vi "Replace-PointOnBody-Dimension.vi"(6 "Add?":bool, 8 "Dimension":dbl, 9 "DimensionIndex":i32, 11 "Point":T1={"Coord4"=[0.0, 0.0, 0.0, 1.0], "ID"=0}) -> (3 "Point 2":T1={"Coord4"=[0.0, 0.0, 0.0, 1.0], "ID"=0})   [LabVIEW 2016, in "CAlex2.lvclass"]
uses:
  CAlex2.lvclass
  SerialChain/TypeDef/PointOnBody.ctl
  SerialChain/SerialChain.lvclass
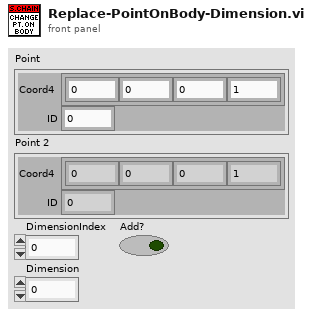
[diagram p1: front panel]
types:
  T1 = typedef "SerialChain.lvclass/PointOnBody.ctl" = cluster{"Coord4":dbl[], "ID":i32}
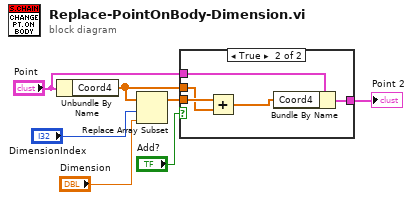
[diagram p0: block diagram]
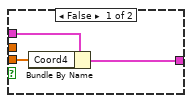
[diagram p2: hidden frame]
diagram:
  n1 = Unbundle By Name("Point") -> ("Coord4"=w1:dbl[])
  n2 = Replace Array Subset(array=w1, new element="Dimension", index="DimensionIndex") -> (w4:dbl[])
  n3 = case shown="True" "Add?" {
    tunnel: w4 -> [w10 w13]
    tunnel: "Point" -> [w9 w15]
    tunnel: [w8 w14] -> w2
    tunnel: w1 -> [_ w12]
    frame False {
      n4 = Bundle By Name(cluster=w9, "Coord4"=w10) -> (w8:T1)
    }
    frame True {
      n5 = Add(x=w13, y=w12) -> (x+y=w11:dbl[])
      n6 = Bundle By Name(cluster=w15, "Coord4"=w11) -> (w14:T1)
    }
  }
  "Point 2" <- w2
